vi "DPOAE Analysis Panel.vi"(9 "Autosave? (F)":bool, 11 "Data folder in":path) -> ()   [LabVIEW 2020]
uses:
  epl-vi-lib/Utility VIs/Controls/KLegend/KLegend.xctl
  Typedefs/DP-Comparison List.ctl
  <vilib>/regexp/Match Regular Expression.xnode
panel:
  out "IOLeg":i32(xcontrol)
  in  "Tab Control":enum32{"Isoresponse", "DP vs F2"}(tab)
  out "DPGram":cluster{"I-O Plot":dbl[], "I-O Plot":dbl[]}[](graph)
  out "DPvsFreq":cluster{"I-O Plot":dbl[], "I-O Plot":dbl[]}[](graph)
  out "DPvsF2Leg":i32(xcontrol)
  out "exit signal":bool
  in  "Save programatically":bool
  in  "Analysis mode":enum32{"Browse", "Compare"}(tab)=enum."Compare"
  in  "Compare>":bool
  in  "File list":i32[](listbox)
  in  "Save":bool
  in  "Data folder":path
  in  "Compare list":i32[](listbox)=[0]
  in  "Criterion (dB SPL)":u16(ring)=1 items=["-5", "0", "5", "10", "15", "20", "25"]
  in  "F2 (kHz)":u16(ring) items=["5645.70", "7995.60", "11322.00", "15991.00", "22644.00", "32012.00", "45257.00", "3997.80", "5615.20", "11291.00", "22613.00"]
  in  "Exit":bool
  out "Noise Floor":i32(listbox)=2
  in  "Which DP":enum16{"2f1-f2", "f2-f1"}(ring)
  out "I-O Plot":cluster{"I-O Plot":dbl[], "I-O Plot":dbl[]}[](graph)
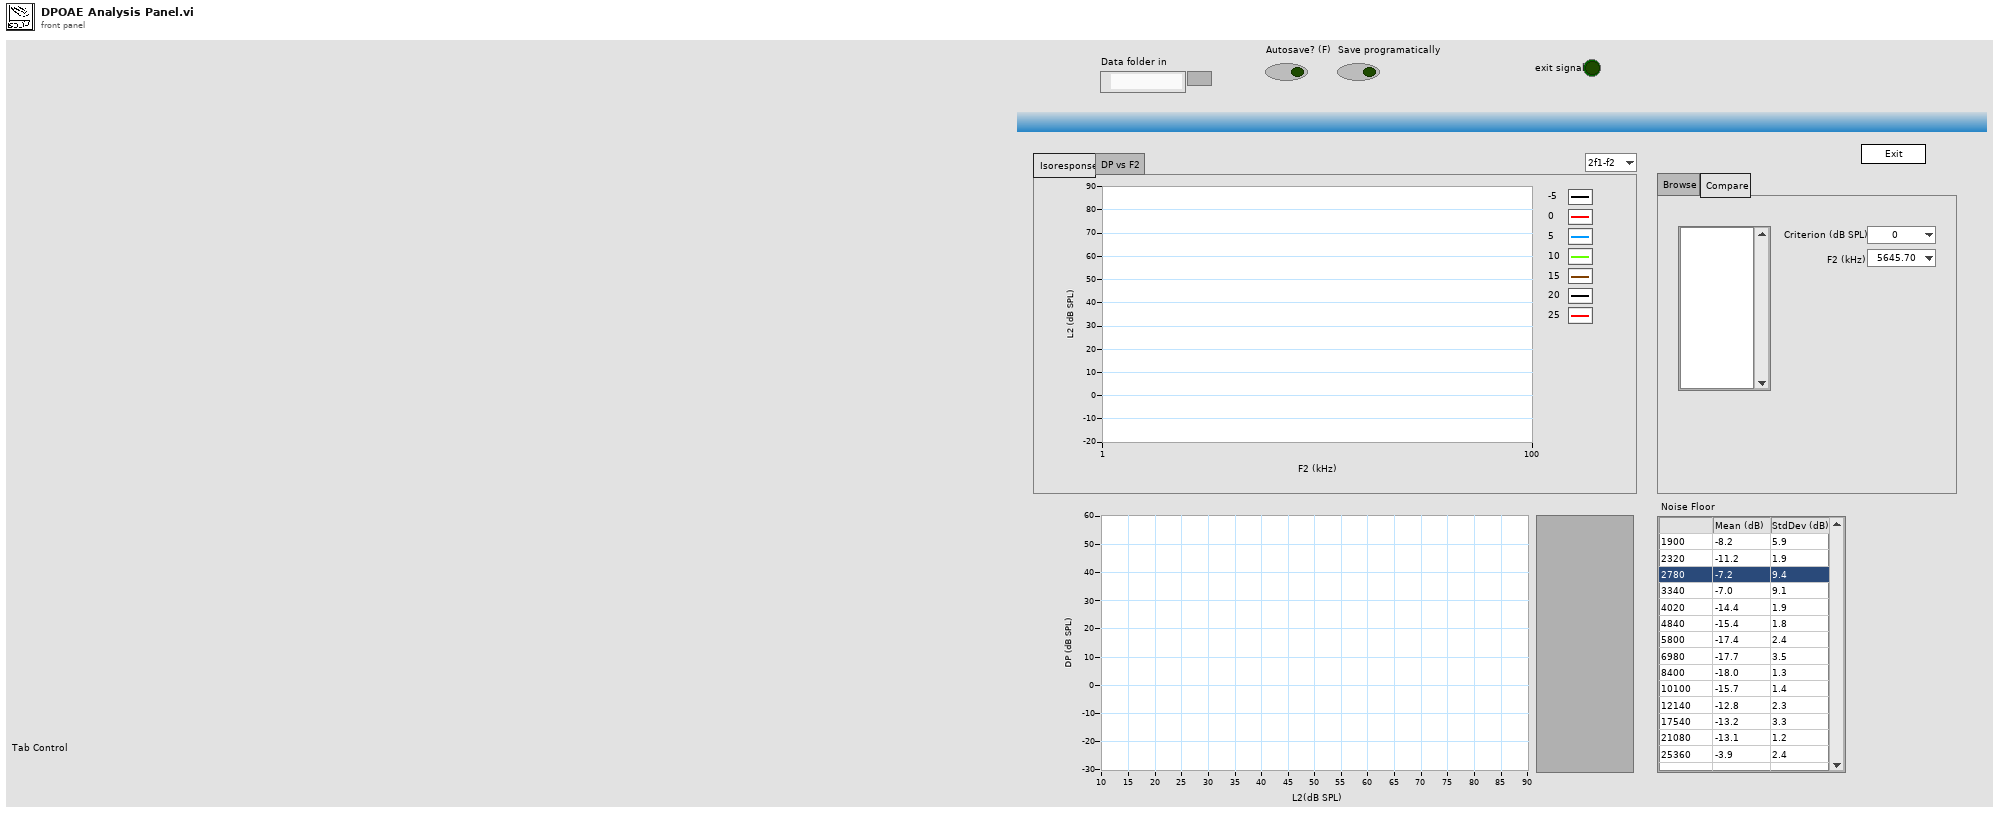
[diagram p1: front panel]
types:
  T1 = typedef "DP-Comparison List.ctl" = cluster{"Name":string, "Path":path, "Show":bool}[]
  T2 = cluster{"Array Subset":dbl[], "Array Subset":dbl[]}[]
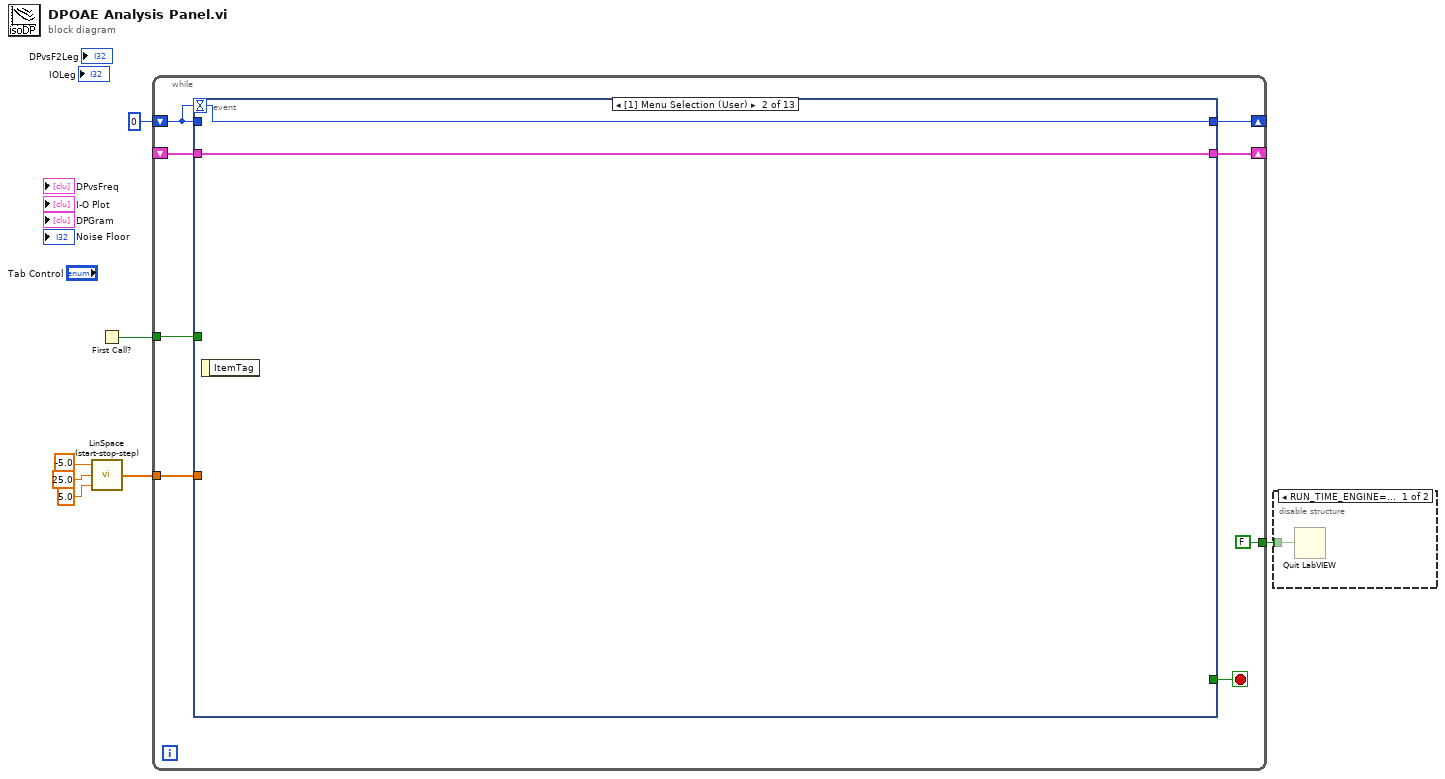
[diagram p0: block diagram]
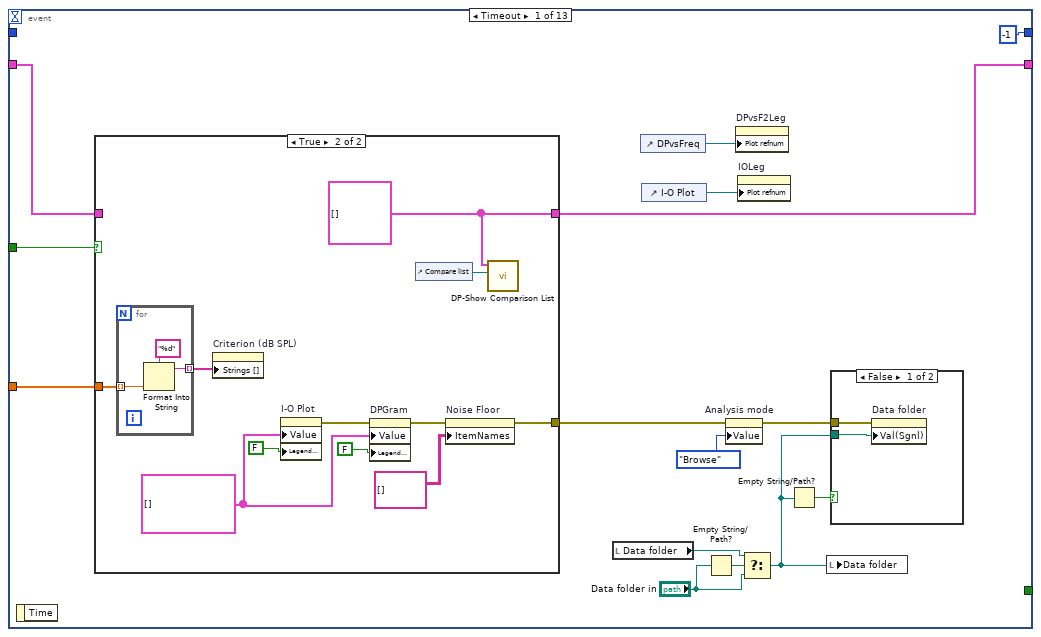
[diagram p3: hidden frame]
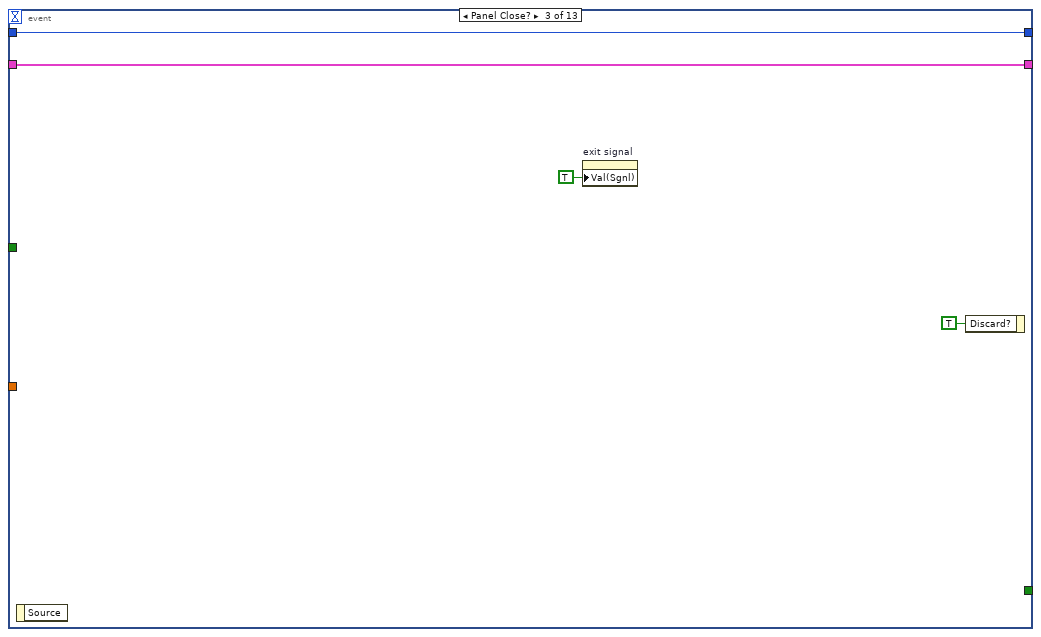
[diagram p6: hidden frame]
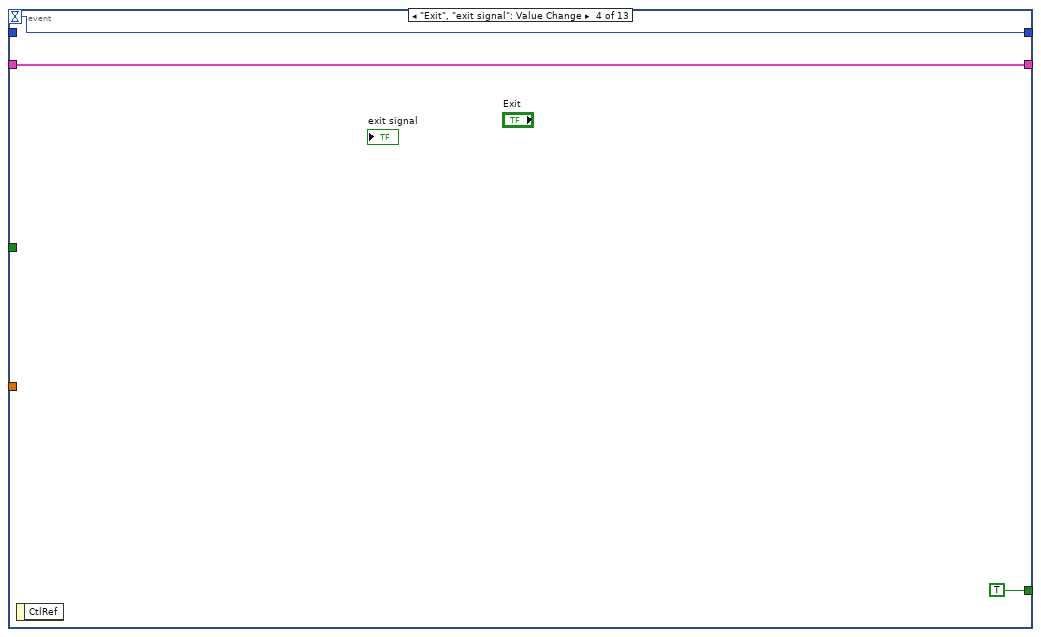
[diagram p7: hidden frame]
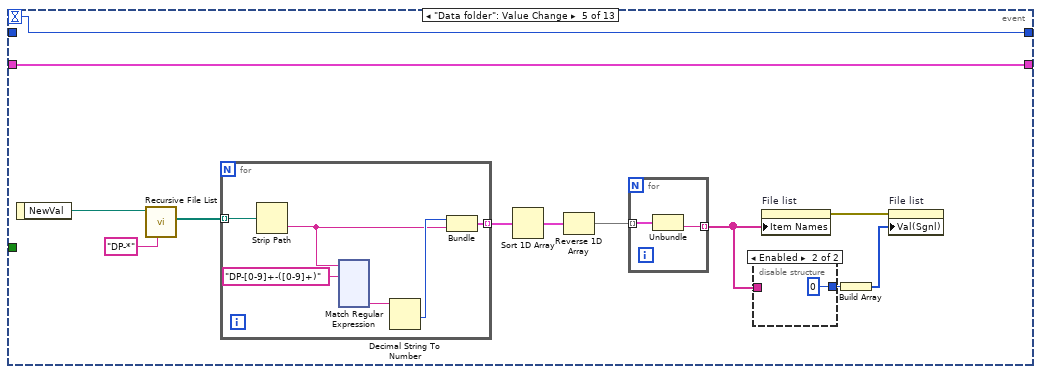
[diagram p8: hidden frame]
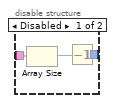
[diagram p9: hidden frame]
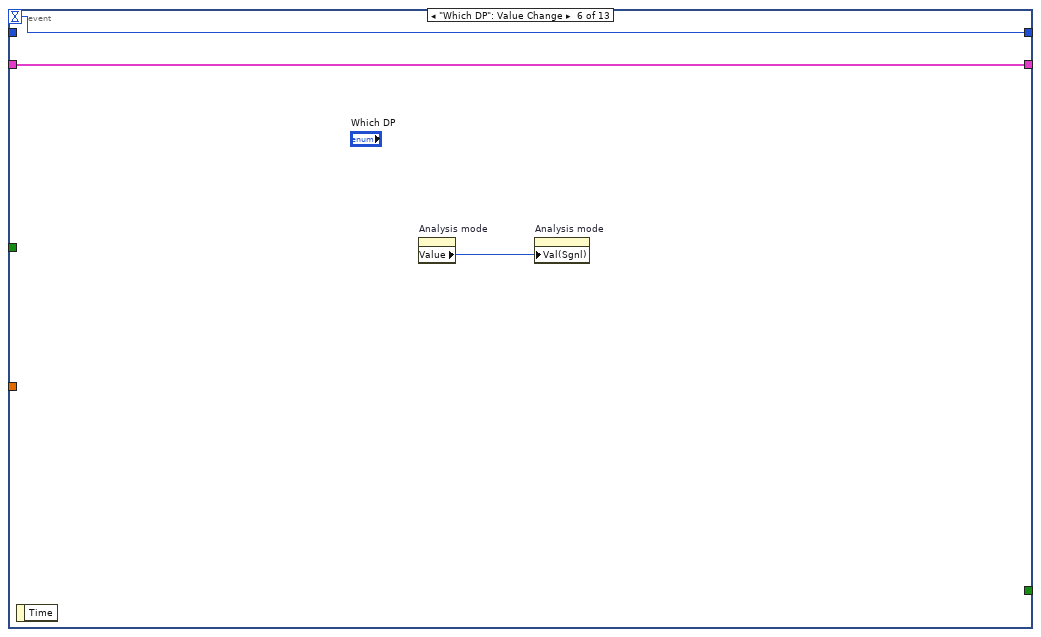
[diagram p10: hidden frame]
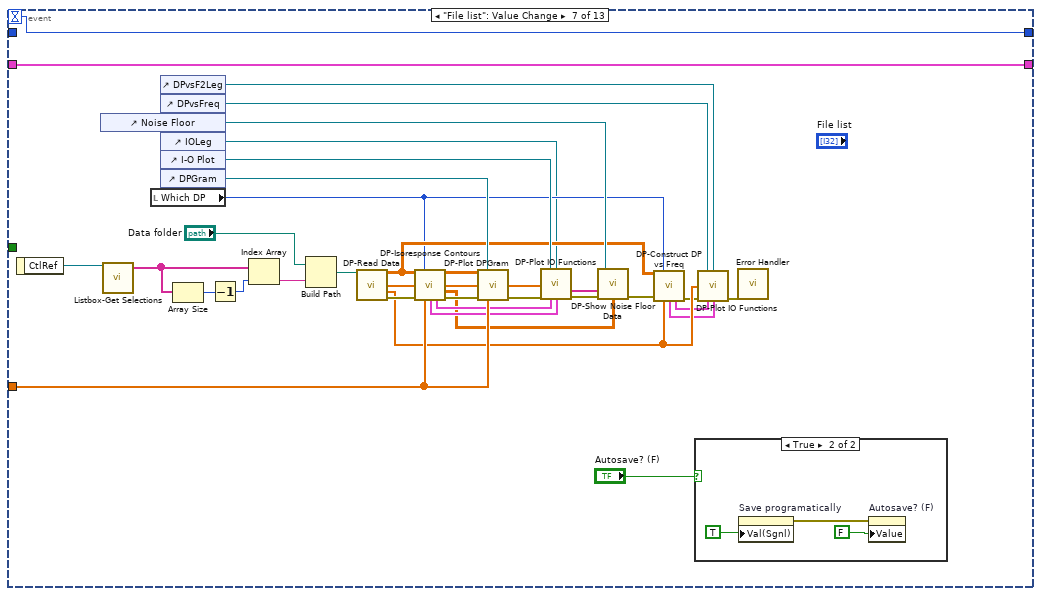
[diagram p11: hidden frame]
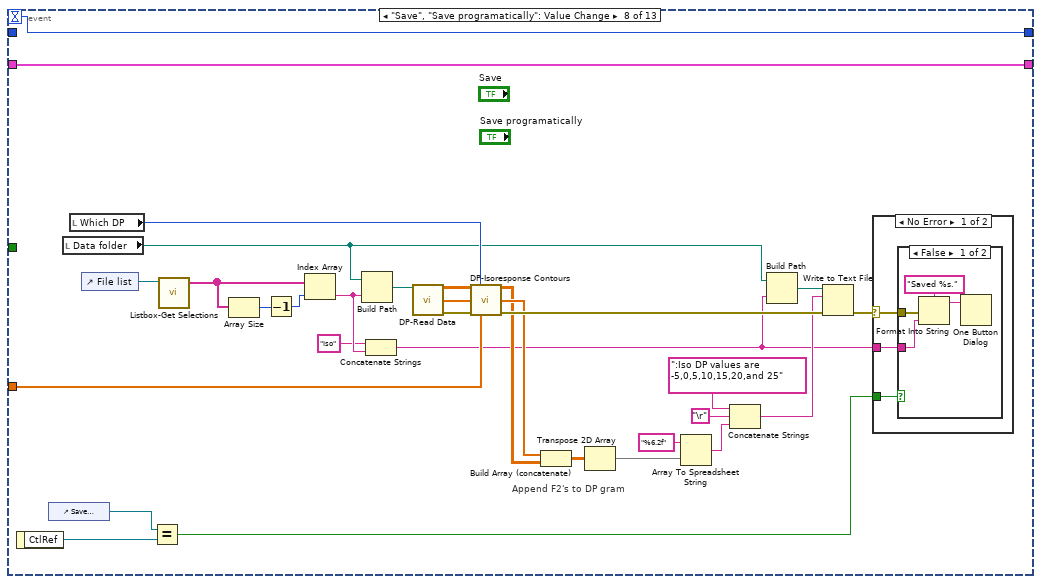
[diagram p13: hidden frame]
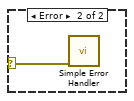
[diagram p15: hidden frame]
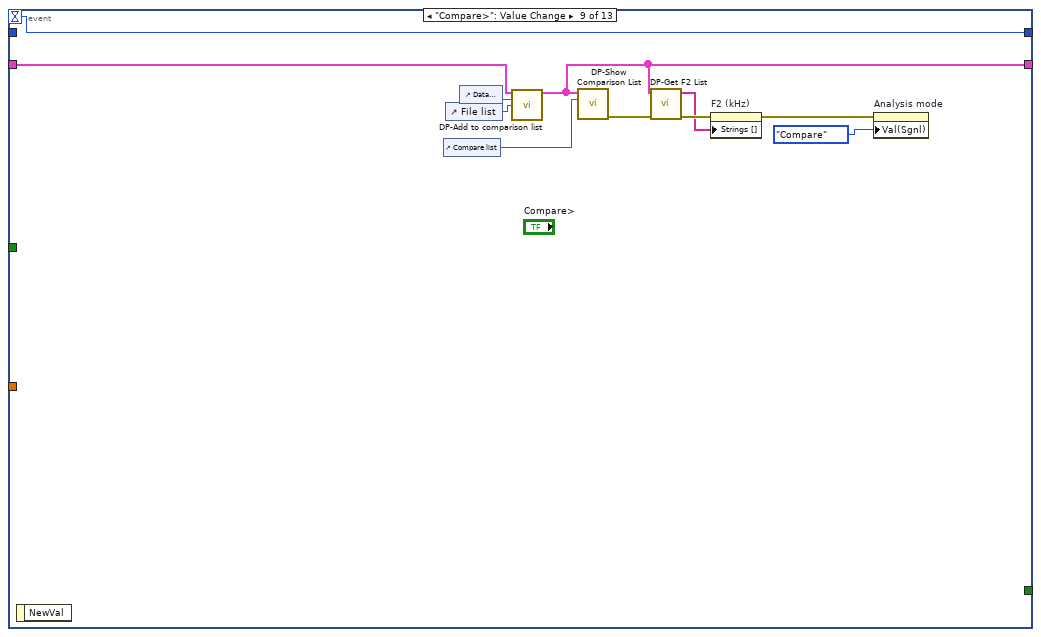
[diagram p16: hidden frame]
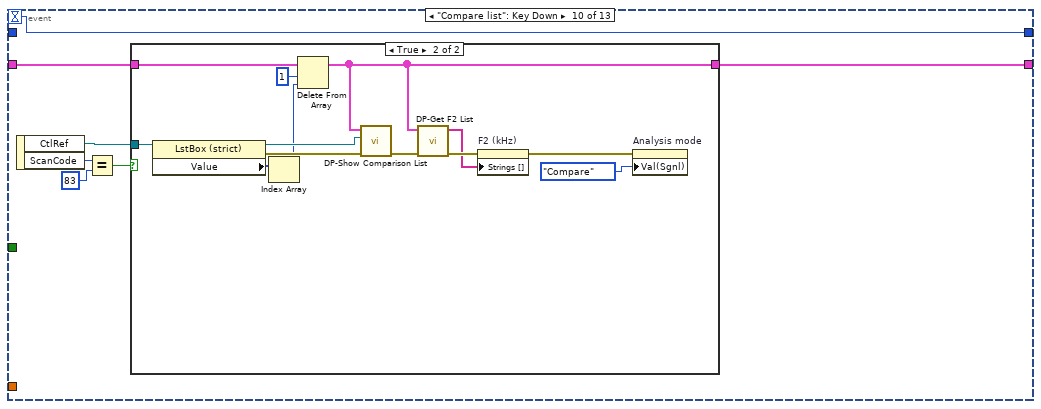
[diagram p17: hidden frame]
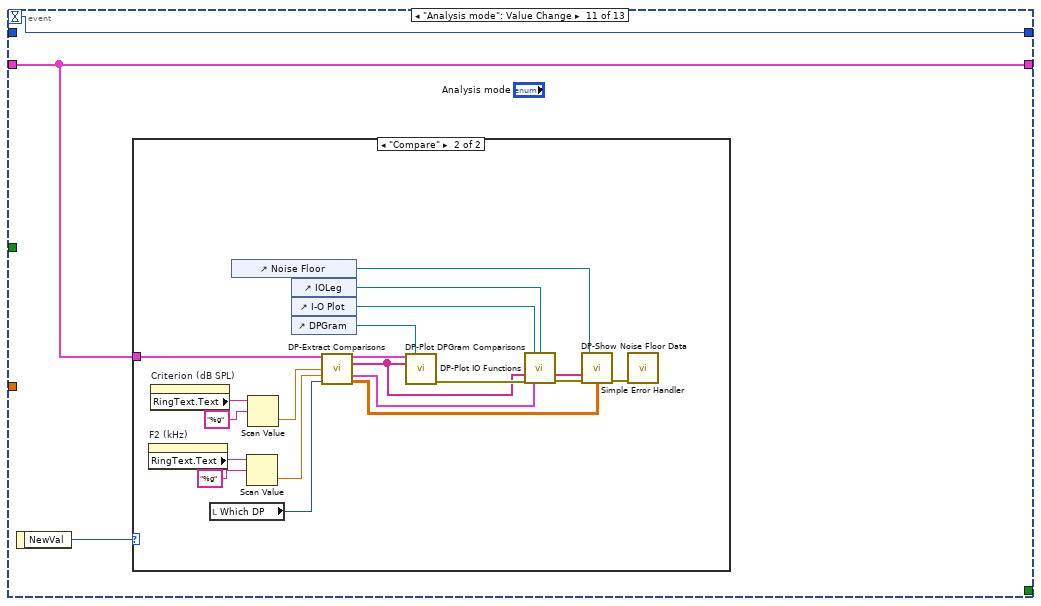
[diagram p19: hidden frame]
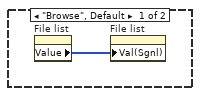
[diagram p20: hidden frame]
diagram:
  n1 = call "LinSpace (start-stop-step).vi"("Step"=5.0, "Stop"=25.0, "Start"=-5.0) -> ("Array"=w2:dbl[])  [unwired: 1 in, 1 out]
  n2 = First Call?() -> (First Call?: T/F=w6:bool)
  n3 = while {
    shift-right: [w14] -> _
    shift-left: 0 -> [w9]
    tunnel: w6 -> [w13]
    tunnel: w2 -> [w12]
    shift-right: [w11] -> _
    shift-left: _ -> [w10]
    tunnel: [FALSE] -> w1
    stop <- w15 stop-if-true
    n4 = event shown="[1] Menu Selection (User)" {
      selector: _ -> [_ _ _ _ _ _ _ _ _ _ _ _ _]
      dyn-events: _ -> [_ _ _ _ _ _ _ _ _ _ _ _ _]
      timeout: w9 -> [_ w49 _ w55 w68 w199 w236 w270 w288 w296 w313 w337 w348]
      tunnel: [_ _ _ TRUE _ _ _ _ _ _ _ _ _] -> w15
      tunnel: [-1 w49 w51 w55 w68 w199 w236 w270 w288 w296 w313 w337 w348] -> w14
      tunnel: w13 -> [w29 _ _ _ _ _ _ _ _ _ _ _ _]
      tunnel: w12 -> [w28 _ _ _ _ _ w231 w245 _ _ _ _ _]
      tunnel: [w27 w48 w52 w54 w64 w198 w217 w269 w281 w291 w311 w336 w340] -> w11
      tunnel: w10 -> [w26 w48 w52 w54 w64 w198 w217 w269 w279 w292 w311 w336 w344]
      tunnel: w9 -> [_ _ w51 _ _ _ _ _ _ _ _ _ _]
      event Timeout {
        n5 = event-data() -> ()  [unwired: 1 in, 1 out]
        n6 = case shown="True" w29 {
          tunnel: w28 -> [_ w38]
          tunnel: [w33 w35] -> w27
          tunnel: w26 -> [w33 _]
          tunnel: [_ w34] -> w18
          frame False {
          }
          frame True {
            w35 = T1 [] ("Comparison list")
            w42 = cluster{"I-O Plot":dbl[], "I-O Plot":dbl[]}[] [] ("I-O Plot")
            n7 = for {
              tunnel: w38 -> [w46] mode=indexing
              tunnel: [w47] -> w37 mode=indexing
              n8 = Format Into String(format string="%d", w46) -> (resulting string=w47:string)  [unwired: 2 in, 1 out]
            }
            n9 = property on="Criterion (dB SPL)" class="Ring (strict)"("Strings []"=w37) -> ()  [unwired: 2 in, 2 out]
            n10 = property on="I-O Plot" class="XYGraph (strict)"("Value"=w42, "Legend Visible"=FALSE ("Legend:Visible")) -> (error out=w43:errorcluster)  [unwired: 2 in, 1 out]
            n11 = property on="DPGram" class="XYGraph (strict)"(error in=w43, "Value"=w42, "Legend Visible"=FALSE ("Legend:Visible")) -> (error out=w40:errorcluster)  [unwired: 1 in, 1 out]
            n12 = control-ref of="Compare list"() -> (w36:refnum<vi>)
            n13 = property on="Noise Floor" class="MCListbox (strict)"(error in=w40, "ItemNames"=string[][] [] ("Item Names")) -> (error out=w34:errorcluster)  [unwired: 1 in, 1 out]
            n14 = call "DP-Show Comparison List.vi"("Listbox Ref"=w36, "Comparison list"=w35) -> ()  [unwired: 9 in, 1 out]
          }
        }
        n15 = local read "Data folder"() -> (w24:path)
        n16 = control-ref of="DPvsFreq"() -> (w17:refnum<vi>)
        n17 = control-ref of="I-O Plot"() -> (w16:refnum<vi>)
        n18 = Empty String/Path?(string/path="Data folder in") -> (empty?=w22:bool)
        n19 = property on="Analysis mode" class="TabCtl (strict)"(error in=w18, "Value"=enum32{"Browse", "Compare"}."Browse" ("Analysis mode")) -> (error out=w19:errorcluster)  [unwired: 1 in, 1 out]
        n20 = property on="DPvsF2Leg" class="KLegend (strict)"("Plot refnum"=w17) -> ()  [unwired: 2 in, 2 out]
        n21 = property on="IOLeg" class="KLegend (strict)"("Plot refnum"=w16) -> ()  [unwired: 2 in, 2 out]
        n22 = Select(t=w24, s=w22, f="Data folder in") -> (s? t:f=w25:path)
        n23 = Empty String/Path?(string/path=w25) -> (empty?=w21:bool)
        n24 = local write "Data folder"(w25) -> ()
        n25 = case shown="False" w21 {
          tunnel: w25 -> [w32 _]
          tunnel: w19 -> [w31 _]
          frame False {
            n26 = property on="Data folder" class="Path"(error in=w31, "Val(Sgnl)"=w32) -> ()  [unwired: 1 in, 2 out]
          }
          frame True {
          }
        }
      }
      event Menu Selection (User) {
        n27 = event-data() -> ()  [unwired: 1 in, 1 out]
      }
      event Panel Close? {
        n28 = event-data() -> ()  [unwired: 1 in, 1 out]
        n29 = property on="exit signal" class="Bool (strict)"("Val(Sgnl)"=TRUE ("Value (Signaling)")) -> ()  [unwired: 2 in, 2 out]
        n30 = event-data("Discard?"=TRUE) -> ()  [unwired: 1 in, 1 out]
      }
      event "Exit", "exit signal": Value Change {
        n31 = event-data() -> ()  [unwired: 1 in, 1 out]
      }
      event "Data folder": Value Change {
        n32 = event-data() -> ("NewVal"=w67:path)  [unwired: 1 in]
        n33 = call <vilib>:"Recursive File List.vi"("pattern"="DP-*", "Folder Path"=w67) -> ("All Files in Dir"=w65:path[])  [unwired: 5 in, 4 out]
        n34 = for {
          tunnel: w65 -> [w80] mode=indexing
          tunnel: [w77] -> w60 mode=indexing
          n35 = Strip Path(path=w80) -> (name=w75:string)  [unwired: 1 out]
          n36 = xnode "Match Regular Expression"("input string"=w75, "regular expression"="DP-[0-9]+-([0-9]+)") -> ("submatch 1"=w78:string)  [unwired: 4 in, 5 out]
          n37 = Decimal String To Number(string=w78) -> (number=w76:i32)  [unwired: 2 in, 1 out]
          n38 = Bundle(w76, "name"=w75) -> (w77:cluster{i32, "name":string})  [unwired: 1 in]
        }
        n39 = Sort 1D Array(array=w60) -> (sorted array=w59:cluster{i32, "name":string}[])
        n40 = Reverse 1D Array(array=w59) -> (reversed array=w57:cluster{i32, "name":string}[])
        n41 = for {
          tunnel: w57 -> [w74] mode=indexing
          tunnel: [w73] -> w58 mode=indexing
          n42 = Unbundle(w74) -> ("name"=w73:string)  [unwired: 1 out]
        }
        n43 = disable-structure shown="Enabled" {
          disable-tunnel: [w70 0] -> w62
          disable-tunnel: w58 -> [w69 _]
          frame Disabled {
            n44 = Array Size(array=w69) -> (size(s)=w71:i32)
            n45 = Decrement(x=w71) -> (x-1=w70:i32)
          }
          frame Enabled {
          }
        }
        n46 = property on="File list" class="LstBox (strict)"("Item Names"=w58) -> (error out=w63:errorcluster)  [unwired: 2 in, 1 out]
        n47 = Build Array(w62) -> (w61:i32[])
        n48 = property on="File list" class="LstBox (strict)"(error in=w63, "Val(Sgnl)"=w61) -> ()  [unwired: 1 in, 2 out]
      }
      event "Which DP": Value Change {
        n49 = event-data() -> ()  [unwired: 1 in, 1 out]
        n50 = property on="Analysis mode" class="TabCtl (strict)"() -> ("Value"=w197:enum32{"Browse", "Compare"})  [unwired: 2 in, 2 out]
        n51 = property on="Analysis mode" class="TabCtl (strict)"("Val(Sgnl)"=w197) -> ()  [unwired: 2 in, 2 out]
      }
      event "File list": Value Change {
        n52 = event-data() -> ("CtlRef"=w216:refnum<vi>)  [unwired: 1 in]
        n53 = control-ref of="Noise Floor"() -> (w233:refnum<vi>)
        n54 = call "Listbox-Get Selections.vi"("Listbox Ref"=w216) -> ("Selections"=w230:string[])  [unwired: 9 in, 1 out]
        n55 = local read "Which DP"() -> (w211:enum16{"2f1-f2", "f2-f1"})
        n56 = control-ref of="DPvsF2Leg"() -> (w208:refnum<vi>)
        n57 = control-ref of="DPvsFreq"() -> (w210:refnum<vi>)
        n58 = control-ref of="IOLeg"() -> (w207:refnum<vi>)
        n59 = control-ref of="I-O Plot"() -> (w234:refnum<vi>)
        n60 = control-ref of="DPGram"() -> (w235:refnum<vi>)
        n61 = Array Size(array=w230) -> (size(s)=w219:i32)
        n62 = Decrement(x=w219) -> (x-1=w218:i32)
        n63 = Index Array(array=w230, index=w218) -> (element=w221:string)
        n64 = Build Path(base path="Data folder", name or relative path=w221) -> (appended path=w220:path)
        n65 = call "DP-Read Data.vi"("Path"=w220) -> ("Data matrix"=w212:dbl[][], "F2 array"=w213:dbl[], "L2 array"=w209:dbl[], "error out"=w229:errorcluster)  [unwired: 11 in]
        n66 = call "DP-Isoresponse Contours.vi"("Data matrix"=w212, "Which DP"=w211, "F2 array"=w213, "error in"=w229, "criteria (dB)"=w231) -> ("DPGram"=w227:dbl[][], "F2 out"=w226:dbl[], "Noise floor data"=w200:dbl[][], "Array"=w201:T2, "IO Functions"=w223:T2, "error out"=w228:errorcluster)  [unwired: 5 in]
        n67 = call "DP-Plot DPGram.vi"("DPGram"=w227, "Plot refnum"=w235, "F2"=w226, "error in"=w228, "criteria (dB)"=w231) -> ("F2 out"=w225:dbl[], "error out"=w224:errorcluster)  [unwired: 8 in, 1 out]
        n68 = call "DP-Plot IO Functions.vi"("Plot refnum"=w234, "Legend"=w207, "Vals"=w225, "error in"=w224, "Value"=w223, "noise"=w201) -> ("Names out"=w206:string[], "error out"=w222:errorcluster)  [unwired: 8 in]
        n69 = call "DP-Show Noise Floor Data.vi"("Listbox Refnum"=w233, "Names"=w206, "error in"=w222, "Noise floor data"=w200) -> ("error out"=w214:errorcluster)  [unwired: 11 in]
        n70 = call "DP-Construct DP vs Freq.vi"("Data matrix"=w212, "Which DP"=w211, "error in"=w214, "L2 array"=w209) -> ("noise floor"=w202:T2, "IO Functions"=w205:T2, "error out"=w204:errorcluster)  [unwired: 9 in]
        n71 = case shown="True" "Autosave? (F)" {
          frame False {
          }
          frame True {
            n72 = property on="Save programatically" class="Bool (strict)"("Val(Sgnl)"=TRUE ("Value (Signaling)")) -> (error out=w238:errorcluster)  [unwired: 2 in, 1 out]
            n73 = property on="Autosave? (F)" class="Bool (strict)"(error in=w238, "Value"=FALSE ("Autosave? (F)")) -> ()  [unwired: 1 in, 2 out]
          }
        }
        n74 = call "DP-Plot IO Functions.vi"("Plot refnum"=w210, "Legend"=w208, "Vals"=w209, "error in"=w204, "Value"=w205, "noise"=w202) -> ("error out"=w203:errorcluster)  [unwired: 8 in, 1 out]
        n75 = call "Error Handler.vi"("error in (no error)"=w203) -> ()  [unwired: 13 in, 2 out]
      }
      event "Save", "Save programatically": Value Change {
        # "Append F2's to DP gram"
        n76 = event-data() -> ("CtlRef"=w241:refnum<vi>)  [unwired: 1 in]
        n77 = control-ref of="Save programatically"() -> (w242:refnum<vi>)
        n78 = local read "Data folder"() -> (w257:path)
        n79 = local read "Which DP"() -> (w261:enum16{"2f1-f2", "f2-f1"})
        n80 = control-ref of="File list"() -> (w260:refnum<vi>)
        n81 = Equal?(x=w242, y=w241) -> (x = y?=w240:bool)
        n82 = call "Listbox-Get Selections.vi"("Listbox Ref"=w260) -> ("Selections"=w268:string[])  [unwired: 9 in, 1 out]
        n83 = Array Size(array=w268) -> (size(s)=w263:i32)
        n84 = Decrement(x=w263) -> (x-1=w262:i32)
        n85 = Index Array(array=w268, index=w262) -> (element=w259:string)
        n86 = Build Path(base path=w257, name or relative path=w259) -> (appended path=w264:path)
        n87 = Concatenate Strings("Iso" ("string"), w259) -> (w243:string)
        n88 = call "DP-Read Data.vi"("Path"=w264) -> ("Data matrix"=w267:dbl[][], "F2 array"=w265:dbl[], "error out"=w266:errorcluster)  [unwired: 11 in, 1 out]
        n89 = call "DP-Isoresponse Contours.vi"("Data matrix"=w267, "Which DP"=w261, "F2 array"=w265, "error in"=w266, "criteria (dB)"=w245) -> ("DPGram"=w248:dbl[][], "F2 out"=w249:dbl[], "error out"=w251:errorcluster)  [unwired: 5 in, 3 out]
        n90 = Build Array (concatenate)(w249, w248) -> (w247:dbl[][])
        n91 = Transpose 2D Array(2D array=w247) -> (transposed array=w246:dbl[][])
        n92 = Array To Spreadsheet String(array=w246, 3:"%6.2f") -> (spreadsheet string=w256:string)  [unwired: 1 in]
        n93 = Concatenate Strings(":Iso DP values are -5,0,5,10,15,20,and 25", "\r", w256) -> (w250:string)
        n94 = Build Path(base path=w257, name or relative path=w243) -> (appended path=w252:path)
        n95 = Write to Text File(file (use dialog)=w252, text=w250, error in=w251) -> (error out=w244:errorcluster)  [unwired: 1 in, 2 out]
        n96 = case shown="No Error" w244 {
          selector: w244 -> [w273 w278]
          tunnel: w243 -> [w272 _]
          tunnel: w240 -> [w271 _]
          frame No Error {
            n97 = case shown="False" w271 {
              tunnel: w273 -> [w277 _]
              tunnel: w272 -> [w274 _]
              frame False {
                n98 = Format Into String(format string="Saved %s.", error in=w277, w274) -> (resulting string=w276:string)  [unwired: 1 in, 1 out]
                n99 = One Button Dialog(message=w276) -> ()  [unwired: 1 in, 1 out]
              }
              frame True {
              }
            }
          }
          frame Error {
            n100 = call <vilib>:"Simple Error Handler.vi"("error in (no error)"=w278) -> ()  [unwired: 4 in, 5 out]
          }
        }
      }
      event "Compare>": Value Change {
        n101 = event-data() -> ()  [unwired: 1 in, 1 out]
        n102 = control-ref of="Compare list"() -> (w282:refnum<vi>)
        n103 = control-ref of="File list"() -> (w287:refnum<vi>)
        n104 = control-ref of="Data folder"() -> (w283:refnum<vi>)
        n105 = call "DP-Add to comparison list.vi"("Comparison list"=w279, "Data folder ref"=w283, "File listbox ref"=w287) -> ("Comparison list out"=w281:T1)  [unwired: 12 in]
        n106 = call "DP-Show Comparison List.vi"("Listbox Ref"=w282, "Comparison list"=w281) -> ("error out"=w286:errorcluster)  [unwired: 9 in]
        n107 = call "DP-Get F2 List.vi"("error in (no error)"=w286, "Comparison list"=w281) -> ("error out"=w289:errorcluster, "F2 List"=w284:string[])  [unwired: 8 in]
        n108 = property on="F2 (kHz)" class="Ring (strict)"(error in=w289, "Strings []"=w284) -> (error out=w280:errorcluster)  [unwired: 1 in, 1 out]
        n109 = property on="Analysis mode" class="TabCtl (strict)"(error in=w280, "Val(Sgnl)"=enum32{"Browse", "Compare"}."Compare" ("Value (Signaling)")) -> ()  [unwired: 1 in, 2 out]
      }
      event "Compare list": Key Down {
        n110 = event-data() -> ("CtlRef"=w290:refnum<vi>, "ScanCode"=w295:i16)  [unwired: 1 in]
        n111 = Equal?(x=w295, y=i16 83) -> (x = y?=w293:bool)
        n112 = case shown="True" w293 {
          tunnel: w292 -> [w297 w310]
          tunnel: [w297 w303] -> w291
          tunnel: w290 -> [_ w302]
          frame False {
          }
          frame True {
            n113 = property class="LstBox (strict)"(reference=w302) -> (reference out=w299:refnum<vi>, error out=w300:errorcluster, "Value"=w301:i32[])  [unwired: 1 in]
            n114 = Index Array(array=w301) -> (element=w298:i32)  [unwired: 1 in]
            n115 = Delete From Array(array=w310, length=1, index=w298) -> (array with subset deleted=w303:T1)  [unwired: 1 out]
            n116 = call "DP-Show Comparison List.vi"("error in (no error)"=w300, "Listbox Ref"=w299, "Comparison list"=w303) -> ("error out"=w307:errorcluster)  [unwired: 8 in]
            n117 = call "DP-Get F2 List.vi"("error in (no error)"=w307, "Comparison list"=w303) -> ("error out"=w308:errorcluster, "F2 List"=w305:string[])  [unwired: 8 in]
            n118 = property on="F2 (kHz)" class="Ring (strict)"(error in=w308, "Strings []"=w305) -> (error out=w304:errorcluster)  [unwired: 1 in, 1 out]
            n119 = property on="Analysis mode" class="TabCtl (strict)"(error in=w304, "Val(Sgnl)"=enum32{"Browse", "Compare"}."Compare" ("Value (Signaling)")) -> ()  [unwired: 1 in, 2 out]
          }
        }
      }
      event "Analysis mode": Value Change {
        n120 = event-data() -> ("NewVal"=w312:enum32{"Browse", "Compare"})  [unwired: 1 in]
        n121 = case shown="\"Compare\"" w312 {
          tunnel: w311 -> [_ w330]
          frame "Browse", Default {
            n122 = property on="File list" class="LstBox (strict)"() -> ("Value"=w314:i32[])  [unwired: 2 in, 2 out]
            n123 = property on="File list" class="LstBox (strict)"("Val(Sgnl)"=w314) -> ()  [unwired: 2 in, 2 out]
          }
          frame "Compare" {
            n124 = property on="F2 (kHz)" class="Ring (strict)"() -> ("RingText.Text"=w323:string)  [unwired: 2 in, 2 out]
            n125 = property on="Criterion (dB SPL)" class="Ring (strict)"() -> ("RingText.Text"=w329:string)  [unwired: 2 in, 2 out]
            n126 = local read "Which DP"() -> (w326:enum16{"2f1-f2", "f2-f1"})
            n127 = control-ref of="Noise Floor"() -> (w332:refnum<vi>)
            n128 = Scan Value(string=w323, format string="%g") -> (value=w322:dbl)  [unwired: 1 in, 1 out]
            n129 = Scan Value(string=w329, format string="%g") -> (value=w327:dbl)  [unwired: 1 in, 1 out]
            n130 = control-ref of="IOLeg"() -> (w316:refnum<vi>)
            n131 = control-ref of="I-O Plot"() -> (w333:refnum<vi>)
            n132 = control-ref of="DPGram"() -> (w334:refnum<vi>)
            n133 = call "DP-Extract Comparisons.vi"("Comparison list"=w330, "Criterion"=w327, "F2 (kHz)"=w322, "Which DP"=w326) -> ("DP Plots"=w325:cluster{"F2 array":dbl[], "DPGram":dbl[]}[], "Names"=w315:string[], "IO Plots"=w320:T2, "Noise floor data"=w318:dbl[][])  [unwired: 8 in]
            n134 = call "DP-Plot DPGram Comparisons.vi"("Plots"=w325, "Plot refnum"=w334, "Names"=w315) -> ("error out"=w331:errorcluster)  [unwired: 12 in]
            n135 = call "DP-Plot IO Functions.vi"("Plot refnum"=w333, "Legend"=w316, "Names in"=w315, "error in"=w331, "Value"=w320) -> ("Names out"=w319:string[], "error out"=w321:errorcluster)  [unwired: 9 in]
            n136 = call "DP-Show Noise Floor Data.vi"("Listbox Refnum"=w332, "Names"=w319, "error in"=w321, "Noise floor data"=w318) -> ("error out"=w317:errorcluster)  [unwired: 11 in]
            n137 = call <vilib>:"Simple Error Handler.vi"("error in (no error)"=w317) -> ()  [unwired: 4 in, 5 out]
          }
        }
      }
      event "F2 (kHz)", "Criterion (dB SPL)": Value Change {
        n138 = event-data() -> ()  [unwired: 1 in, 1 out]
        n139 = property on="Analysis mode" class="TabCtl (strict)"("Val(Sgnl)"=enum32{"Browse", "Compare"}."Compare" ("Value (Signaling)")) -> ()  [unwired: 2 in, 2 out]
      }
      event "Compare list": Double Click {
        n140 = event-data() -> ("Row"=w343:i32, "CtlRef"=w338:refnum<vi>)  [unwired: 1 in]
        n141 = Index Array(array=w344, index=w343) -> (element=w346:cluster{"Name":string, "Path":path, "Show":bool})
        n142 = Unbundle By Name(w346) -> ("Show"=w347:bool)
        n143 = Not(x=w347) -> (.not. x?=w345:bool)
        n144 = Bundle By Name(cluster=w346, "Show"=w345) -> (w342:cluster{"Name":string, "Path":path, "Show":bool})
        n145 = Replace Array Subset(array=w344, new element=w342, index=w343) -> (w340:T1)
        n146 = call "DP-Show Comparison List.vi"("Listbox Ref"=w338, "Comparison list"=w340) -> ("error out"=w339:errorcluster)  [unwired: 9 in]
        n147 = property on="Analysis mode" class="TabCtl (strict)"(error in=w339, "Val(Sgnl)"=enum32{"Browse", "Compare"}."Compare" ("Value (Signaling)")) -> ()  [unwired: 1 in, 2 out]
      }
    }
  }
  n148 = disable-structure shown="RUN_TIME_ENGINE==True" {
    disable-tunnel: w1 -> [w349 _]
    frame condition #0 {
      n149 = Quit LabVIEW(quit? (T)=w349) -> ()
    }
    frame condition #1 (active) {
    }
  }
